vi "Support_ShowFrontPanel.vi"(3 "VI Path":path, 5 "error in (no error)":errorcluster) -> (19 "error out":errorcluster)   [LabVIEW 2009]
doc: "Shows front panel on selected VI."
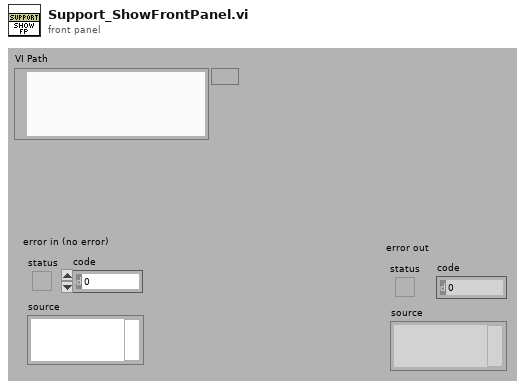
[diagram p1: front panel]
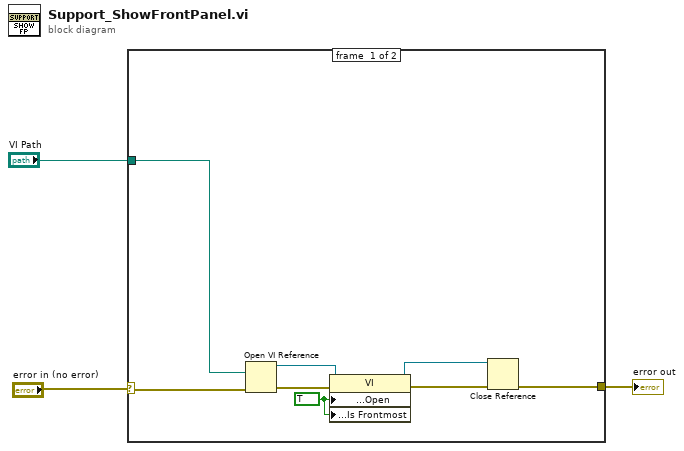
[diagram p0: block diagram]
diagram:
  n1 = case shown="No Error" "error in (no error)" {
    selector: "error in (no error)" -> [w11 w12]
    tunnel: "VI Path" -> [w10 _]
    tunnel: [w6 w12] -> w1
    frame #0 {
      w4 = TRUE ("Front Panel Window:Open")
      n2 = Open VI Reference(vi path=w10, error in (no error)=w11) -> (vi reference=w8:refnum<vi>, error out=w9:errorcluster)  [unwired: 4 in]
      n3 = property class="VI"(reference=w8, error in=w9, "Front Panel Window:Open"=w4, "Front Panel Window:Is Frontmost"=w4) -> (reference out=w5:refnum<vi>, error out=w7:errorcluster)
      n4 = Close Reference(reference=w5, error in (no error)=w7) -> (error out=w6:errorcluster)
    }
    frame #1 {
    }
  }
  "error out" <- w1
